vi "Load Settings.vi"(8 "error in (no error)":errorcluster {"code" format="Error %.0f"}, 11 "Parser Settings In":refnum<class "Parser Settings.lvclass">) -> (0 "error out":errorcluster {"code" format="Error %.0f"}, 3 "Parser Settings Out":refnum<class "Parser Settings.lvclass">)   [LabVIEW 2023, in "VIDoc Parsing.lvlib" / "Parser Settings.lvclass"]
uses:
  Parser Settings.lvclass
  C:/projects/DMC/Tooling/Git-Action-Service/Source/Documentation Generation/Settings/VIDoc Settings/VIDoc Settings.lvclass
  VIDoc Settings/VIDoc Settings.lvclass/VIDoc Settings.ctl
  Parser Settings.lvclass/Parser Settings.ctl
  VIDoc Settings/Get VIDoc Settings Path.vi
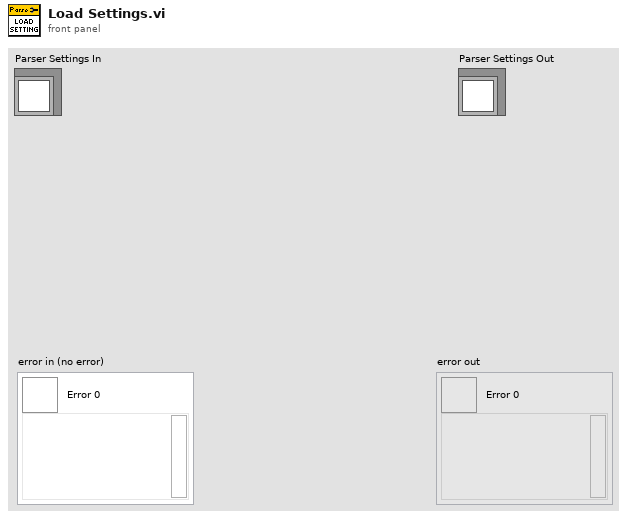
[diagram p1: front panel]
types:
  T1 = typedef "VIDoc Parsing.lvlib/Parser Settings.lvclass/Parser Settings Cluster.ctl" = cluster{"Draw Controls":T2, "Max Control Recursion Depth":i32, "UI Bookmarks":string[], "Subpanel Bookmarks":string[], "Dialog Bookmarks":string[]}
  T2 = typedef "VIDoc Parsing.lvlib/Parser Settings.lvclass/Draw Controls Cluster.ctl" = cluster{"Subpanels":bool, "Tabs":bool, "TypeDefs":bool, "Error Clusters":T3, "DVRs":T3, "Queues & Notifiers":T3}
  T3 = typedef "VIDoc Parsing.lvlib/Parser Settings.lvclass/Draw Option Enum.ctl" = enum16{"Ignore", "Draw", "Draw + Contents"}
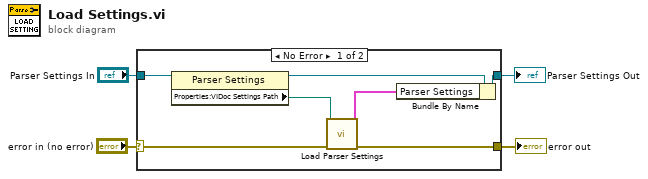
[diagram p0: block diagram]
diagram:
  n1 = case shown="No Error" "error in (no error)" {
    selector: "error in (no error)" -> [w11 w13]
    tunnel: [w10 w13] -> w3
    tunnel: [w6 w12] -> w2
    tunnel: "Parser Settings In" -> [w9 w12]
    frame No Error {
      n2 = property class="Parser Settings"(reference=w9) -> (reference out=w8:refnum<class "Parser Settings.lvclass">, "Properties:VIDoc Settings Path"=w7:path)  [unwired: 1 in, 1 out]
      n3 = call "Load Parser Settings.vi"("Error in"=w11, "Settings Path"=w7) -> ("Error out"=w10:errorcluster, "Parser Settings"=w5:T1)  [unwired: 7 in, 1 out]
      n4 = Bundle By Name(cluster=w8, "Parser Settings"=w5) -> (w6:refnum<class "Parser Settings.lvclass">)
    }
    frame Error {
    }
  }
  "error out" <- w3
  "Parser Settings Out" <- w2
